vi "GetDisplayContentScale.vi"(8 "No Error":errorcluster, 11 "DisplayID":T1) -> (0 "Error Out":errorcluster, 3 "Display Scale":sgl)   [LabVIEW 2024, in "SDL3.lvlib" / "Video.lvlib"]
doc: "<B>Summary</B>\nGet the content display scale relative to a window's pixel size.\n\n<B>Remarks</B>\nThis is a combination of the window pixel density and the display content scale, and is the expected scale for displaying content in this window. For example, if a 3840x2160 window had a display scale of 2.0, the user expects the content to take twice as many pixels and be the same physical size as if it were being displayed in a 1920x1080 window with a display scale of 1.0.\n\nConceptually this value corresponds to the scale display setting, and is updated when that setting is changed, or the window moves to a display with a different scale setting.\n\nNote: This function may fail on systems where the window has not yet been decorated by the display server (for example, immediately after calling SDL_CreateWindow). It is recommended that you wait at least until the window has been presented and composited, so that the window system has a chance to decorate the window and provide the border dimensions to SDL.\n\nThis function also returns false if getting the information is not supported."
uses:
  Video.lvlib
  DisplayID--integer.ctl
  <vilib>/Utility/error.llb/Error Cluster From Error Code.vi
  Lib/SDL3-32.dll
  Error/Error.lvlib
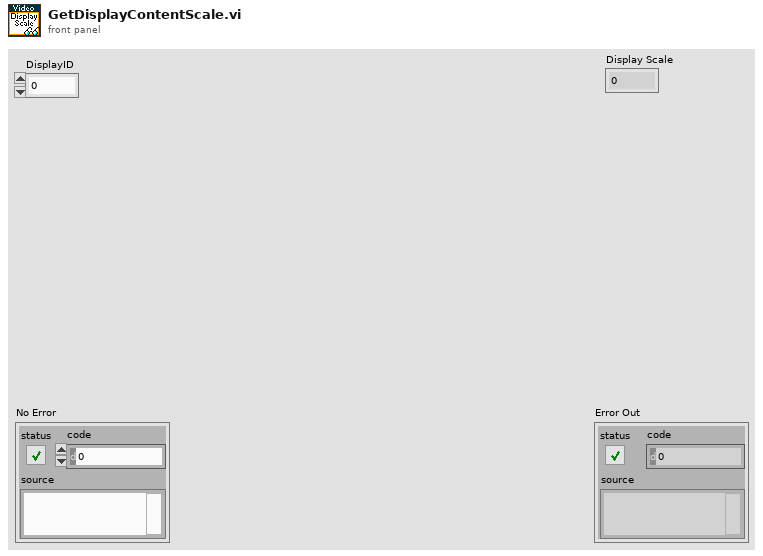
[diagram p1: front panel]
types:
  T1 = typedef "SDL3.lvlib/Video.lvlib/DisplayID--integer.ctl" = u32
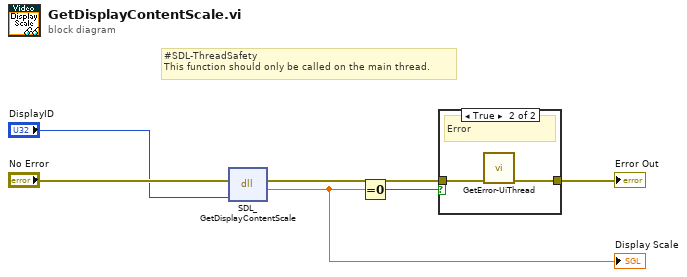
[diagram p0: block diagram]
diagram:
  # "#SDL-ThreadSafety\nThis function should only be called on the main thread."
  n1 = dll-call lib="C:/Users/Thomas/Documents/Projects/LV-SDL3/Lib/SDL3-*.*" fn="SDL_GetDisplayContentScale"(error in="No Error", "displayID"="DisplayID") -> (error out=w3:errorcluster, "return type"=w4:sgl)  [unwired: 3 in, 1 out]
  "Display Scale" <- w4
  n2 = Equal To 0?(x=w4) -> (x = 0?=w2:bool)
  n3 = case shown="True" w2 {
    tunnel: w3 -> [w7 w9]
    tunnel: [w7 w8] -> w5
    frame False {
      # "Ok"
    }
    frame True {
      # "Error"
      n4 = call "GetError-UiThread.vi"("No Error"=w9) -> ("error out"=w8:errorcluster)  [unwired: 10 in]
    }
  }
  "Error Out" <- w5
